vi "labview_fft_tutorial.vi"() -> ()   [LabVIEW 2022 SP3]
uses:
  <vilib>/Analysis/4window.llb/windowTd.ctl
  <vilib>/Analysis/2dsp.llb/Real FFT.vi
  <vilib>/Analysis/0measdsp.llb/Scaled Time Domain Window (DBL).vi
  <vilib>/express/express analysis/Spectral/XNode/ExpressSpectralMeasurementsBlockNode.xnode
  <vilib>/Analysis/NI_AALPro.lvlib
  <vilib>/express/express analysis/Spectral/Block/exnSpectralBlock spectral measurements power poly.vi
  <vilib>/express/express analysis/Spectral/Block/exnSpectralBlock spectral measurements power DDT.vi
panel:
  in  "window":T1 items=["Rectangle"=0, "Hanning"=1, "Hamming"=2, "Blackman-Harris"=3, "Exact Blackman"=4, "Blackman"=5, "Flat Top"=6, "4 Term B-Harris "=7, "7 Term B-Harris"=8, "Low Sidelobe"=9, "Blackman Nuttall"=11, "Triangle"=30, "Bartlett-Hanning"=31, "Bohman"=32, "Parzen"=33, "Welch"=34, "Kaiser"=60, "Dolph-Chebyshev"=61, "Gaussian"=62]
  in  "Samples/s (Hz)":dbl
  in  "FFT size":dbl
  in  "Amplitude":dbl=4.0
  in  "Frequency":dbl=250.0
  out "Waveform Graph 2":dbl[][](graph)
  out "Waveform Graph":dbl[](graph)
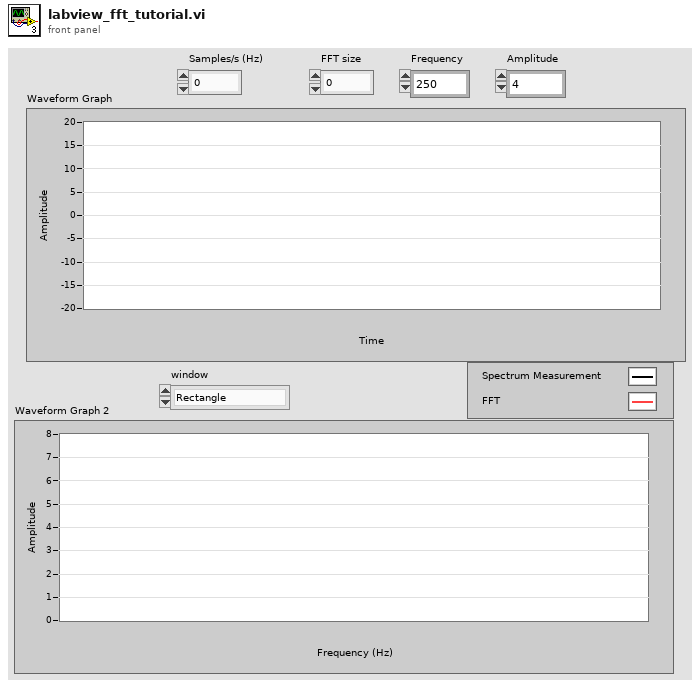
[diagram p1: front panel]
types:
  T1 = typedef "NI_AALPro.lvlib/windowTd.ctl" = u32
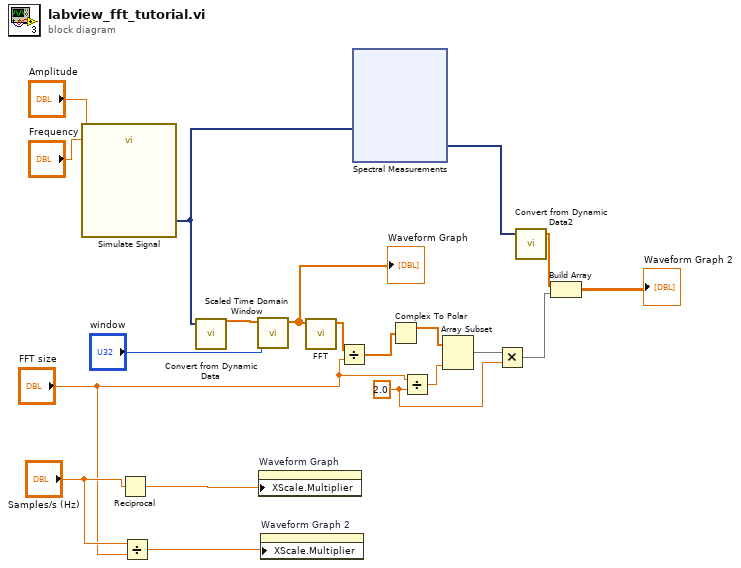
[diagram p0: block diagram]
diagram:
  w9 = 2.0 ("y")
  n1 = call "Simulate Signal"("Frequency"="Frequency", "Amplitude"="Amplitude") -> ("Sine"=w20:dynamicdata)  [unwired: 12 in, 1 out]
  n2 = Reciprocal(x="Samples/s (Hz)") -> (1/x=w7:dbl)
  n3 = Divide(x="Samples/s (Hz)", y="FFT size") -> (x/y=w4:dbl)
  n4 = call "Convert from Dynamic Data"("Dynamic Data Type"=w20) -> ("Array"=w2:dbl[])  [unwired: 3 in]
  n5 = call-poly <vilib>:"Scaled Time Domain Window.vi"("window"="window", "X"=w2) -> ("Windowed X"=w1:dbl[])  [unwired: 7 in, 2 out]
  "Waveform Graph" <- w1
  n6 = property on="Waveform Graph" class="WFGraph (strict)"("XScale.Multiplier"=w7) -> ()  [unwired: 2 in, 2 out]
  n7 = property on="Waveform Graph 2" class="WFGraph (strict)"("XScale.Multiplier"=w4) -> ()  [unwired: 2 in, 2 out]
  n8 = call-poly <vilib>:"FFT.vi"("X"=w1) -> ("FFT {X}"=w14:cdb[])  [unwired: 9 in, 1 out]
  n9 = Divide(x=w14, y="FFT size") -> (x/y=w13:cdb[])
  n10 = xnode "Spectral Measurements"("Signals"=w20) -> ("Power Spectrum"=w19:dynamicdata)  [unwired: 1 in, 1 out]
  n11 = Complex To Polar(r * e^(i*theta)=w13) -> (r=w12:dbl[])  [unwired: 1 out]
  n12 = Divide(x="FFT size", y=w9) -> (x/y=w11:dbl)
  n13 = Array Subset(array=w12, length=w11) -> (w10:dbl[])  [unwired: 1 in]
  n14 = Multiply(x=w10, y=w9) -> (x*y=w8:dbl[])
  n15 = call "Convert from Dynamic Data2"("Dynamic Data Type"=w19) -> ("Array"=w18:dbl[])  [unwired: 3 in]
  n16 = Build Array(w18, w8) -> (→"Waveform Graph 2":dbl[][])
